vi "Post-Object Terminate.vi"(8 "error in (no error)":errorcluster, 11 "Asylum_Driver in":refnum<class "Asylum_Driver.lvclass">) -> (0 "error out":errorcluster, 3 "Asylum_Driver out":refnum<class "Asylum_Driver.lvclass">)   [LabVIEW 2019, in "Asylum_Driver.lvclass"]
uses:
  Asylum_Driver.lvclass
  AFM Driver/AFM_Driver.lvclass
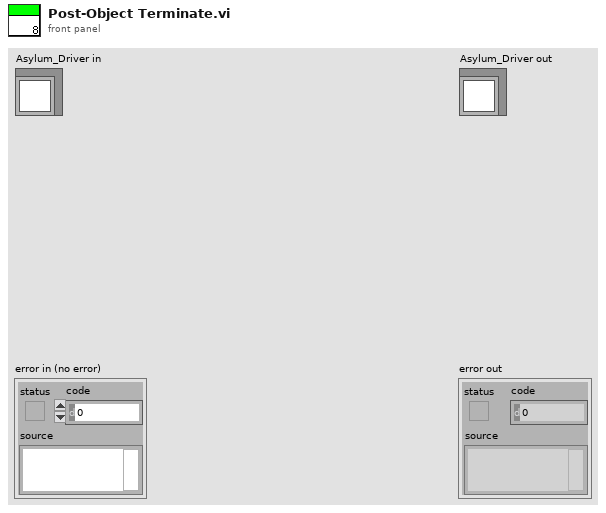
[diagram p1: front panel]
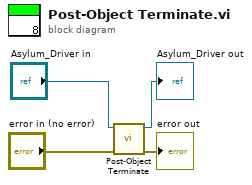
[diagram p0: block diagram]
diagram:
  n1 = call-parent "Post-Object Terminate.vi"("error in (no error)"="error in (no error)", "AFM_Driver in"="Asylum_Driver in") -> ("error out"=→"error out":errorcluster, "AFM_Driver out"=→"Asylum_Driver out":refnum<class "Asylum_Driver.lvclass">)  [unwired: 8 in]
